vi "Running.vi"(8 "error in (no error)":errorcluster, 11 "CIFTemplatePlugin in":refnum<class "TemplatePlugin.lvclass">) -> (0 "error out":errorcluster, 2 "Destroy":bool, 3 "CIFTemplatePlugin out":refnum<class "TemplatePlugin.lvclass">)   [LabVIEW 2021, in "TemplatePlugin.lvclass"]
uses:
  TemplatePlugin.lvclass
  D:/dev/CIF-LVCore/src/CIFCore/Class/CIFCorePlugin.lvclass
  CIF-LVCore/src/CIFCore/Class/CIFCorePlugin.lvclass/CIFCorePlugin.ctl
  TemplatePlugin.lvclass/TemplatePlugin.ctl
  <vilib>/CIF Foundation/CIF Utilities/Statistics/I64/Stats_I64_CIF_U.lvclass/Stats_I64_CIF_U.ctl
  <vilib>/CIF Foundation/CIF Out of Band Commands/CIFOutOfBand.lvclass/CIFOutOfBand.ctl
  CIF-LVCore/src/Channels/CIFChannelMng/CIFChannelMng.lvclass/CIFChannelMng.ctl
  CIF-LVCore/src/CIFCore/OOB/OOB_Rx/CIFCoreOOB_Rx.lvclass/CIFCoreOOB_Rx.ctl
  <vilib>/CIF Foundation/CIF Channels Core/CIFChannels/CIFChannels.lvclass/CIFChannels.ctl
  CIF-LVCore/src/CIFCore/Class/Typedef/Energized States.ctl
  Logic.vi
  CIF-LVCore/src/CIFCore/Class/Accessors/Write Energized State.vi
  CIF-LVCore/src/CIFCore/Class/SubVIs/Sleep.vi
  CIF-LVCore/src/CIFCore/Class/SubVIs/Read Core OOB RX.vi
  gRPC/Read gRCP to Main.vi
  gRPC/Send Main to gRPC.vi
  CIF-LVCore/src/CIFCore/Class/SubVIs/OOB/Update Status from Benchmarks.vi
  CIF-LVCore/src/Channels/CIFChannelMng/Core/Send Channel List Update.vi
  <vilib>/CIF Foundation/CIF Utilities/Time/System Time/Sleep Until Future Time.vi
  <vilib>/CIF Foundation/CIF Utilities/Time/System Time/Get System Time.vi
  CIF-LVCore/src/CIFCore/Class/Channel RW/Read U64.vi
  CIF-LVCore/src/CIFCore/Class/Channel RW/Write U64.vi
  CIF-LVCore/src/CIFCore/Class/Channel RW/Read U8 Array FIFO.vi
  CIF-LVCore/src/CIFCore/Class/Channel RW/Write U8 Array FIFO.vi
  CIF-LVCore/src/CIFCore/Class/Channel RW/Write Double.vi
  CIF-LVCore/src/CIFCore/Class/Channel RW/Read Double.vi
  CIF-LVCore/src/CIFCore/Class/Accessors/Monitor/Write Double 1.vi
  CIF-LVCore/src/CIFCore/Class/Accessors/Monitor/Write U64 1.vi
  CIF-LVCore/src/CIFCore/Class/Accessors/Monitor/Write U64 2.vi
  CIF-LVCore/src/CIFCore/Class/Accessors/Monitor/Write I64 1.vi
  CIF-LVCore/src/CIFCore/Class/Accessors/Monitor/Write I64 2.vi
  CIF-LVCore/src/CIFCore/Class/Accessors/Timestamps/Write Execute TS.vi
  CIF-LVCore/src/CIFCore/Class/Accessors/Timestamps/Write Sleep TS.vi
  <vilib>/Utility/error.llb/Clear Errors.vi
  CIF-LVCore/src/CIFCore/Class/Accessors/Read Sleep Limits (ns).vi
  CIF-LVCore/src/CIFCore/Class/Accessors/Timestamps/Write Target Wake TS.vi
  CIF-LVCore/src/CIFCore/Common/Utilities/Add Error.vi
  CIF-LVCore/src/CIFCore/Class/Accessors/Read Plugin Name.vi
  CIF-LVCore/src/CIFCore/Class/Accessors/Timestamps/Read Running TS.vi
  CIF-LVCore/src/CIFCore/Class/Accessors/Read Running Internal Data.vi
  CIF-LVCore/src/CIFCore/Class/Accessors/Read Timing Override.vi
  CIF-LVCore/src/CIFCore/Class/Accessors/Read Common Config.vi
  CIF-LVCore/src/CIFCore/Class/Accessors/Timestamps/Write Housekeeping TS.vi
  <vilib>/CIF Foundation/CIF Utilities/Statistics/I64/X1 minus X0.vi
  <vilib>/CIF Foundation/CIF Utilities/Statistics/I64/Cyclic.vi
  CIF-LVCore/src/CIFCore/Class/Accessors/Timestamps/Read Execute TS.vi
  CIF-LVCore/src/CIFCore/Class/Accessors/Timestamps/Read Housekeeping TS.vi
  CIF-LVCore/src/CIFCore/Class/Accessors/Timestamps/Read Sleep TS.vi
  CIF-LVCore/src/CIFCore/Class/Accessors/Timestamps/Read Target Wake TS.vi
  CIF-LVCore/src/CIFCore/Class/SubVIs/Refresh Stats.vi
  CIF-LVCore/src/CIFCore/OOB/OOB_Rx/Receive/Read Clock Map.vi
  CIF-LVCore/src/Channels/CIFChannelMng/SubVIs/Connect Channel.vi
  CIF-LVCore/src/CIFCore/OOB/OOB_Rx/Receive/Read Connections.vi
  CIF-LVCore/src/CIFCore/OOB/OOB_Rx/Receive/Read Forces.vi
  CIF-LVCore/src/Channels/CIFChannelMng/SubVIs/Force Channel.vi
  CIF-LVCore/src/Channels/CIFChannelMng/SubVIs/Add FIFO Publisher.vi
  CIF-LVCore/src/CIFCore/OOB/OOB_Rx/Receive/Read Publisher Instance.vi
  CIF-LVCore/src/Channels/CIFChannelMng/Core/Send Publisher Instance Return.vi
  CIF-LVCore/src/Channels/CIFChannelMng/SubVIs/Remove FIFO Publisher.vi
  CIF-LVCore/src/CIFCore/OOB/OOB_Rx/Receive/Check for OOB Commands.vi
  OOB/OOB_Rx/Receive/Read Data.vi
  OOB/OOB_Rx/Receive/Check for OOB Commands.vi
  OOB/OOB_Tx/Send/Update Data.vi
  <vilib>/CIF Foundation/CIF Out of Band Commands/Commit Commands.vi
  CIF-LVCore/src/CIFCore/Class/Accessors/Read Refresh.vi
  <vilib>/CIF Foundation/CIF Utilities/Statistics/I64/Get Stats.vi
  CIF-LVCore/src/Channels/CIFChannelMng/OOB/OOB_Tx/Send/Update Channel List Command.vi
  <vilib>/CIF Foundation/CIF Utilities/Time/SubVIs/Add Error.vi
  <vilib>/CIF Foundation/CIF Utilities/Time/System Time/LabVIEW Time to TAI Time.vi
  <vilib>/CIF Foundation/CIF Utilities/Errors/Append Error Location.vi
  <vilib>/CIF Foundation/CIF Utilities/Statistics/I64/X1 minus X0.vi/dfabcf33-0dbc-4041-80a5-3dc0c86d2989.vi
  <vilib>/CIF Foundation/CIF Utilities/Statistics/I64/Cyclic.vi/dfabcf33-0dbc-4041-80a5-3dc0c86d2989.vi
  CIF-LVCore/src/CIFCore/OOB/OOB_Rx/Private/Read Payload.vi
  CIF-LVCore/src/Channels/CIFChannelMng/Utilities/Get Channel Index by Name.vi
  <vilib>/CIF Foundation/CIF Channels Core/CIFChannels/Accessors/Read Channel State.vi
  <vilib>/CIF Foundation/CIF Channels Core/CIFChannels/Accessors/Read Tag Forced.vi
  CIF-LVCore/src/Channels/CIFChannelMng/SubVIs/Add Error Channel Manager.vi
  CIF-LVCore/src/Channels/CIFChannelMng/OOB/OOB_Tx/Send/FIFO Publisher Return Command.vi
  CIF-LVCore/src/Channels/CIFChannelMng/SubVIs/Get Original FIFO Channel Name.vi
  <vilib>/CIF Foundation/CIF Out of Band Commands/Read Commands.vi
  CIF-LVCore/src/CIFCore/OOB/OOB_Rx/Private/Command Settings.vi
  OOB/OOB_Rx/Private/Read Payload.vi
  OOB/OOB_Rx/Private/Command Settings.vi
  <vilib>/CIF Foundation/CIF Out of Band Commands/Queue Command.vi
  <vilib>/CIF Foundation/CIF Out of Band Commands/Utilities/Command to Bitwise Command.vi
  <vilib>/CIF Foundation/CIF Out of Band Commands/Accessors/Read Local OOB Data.vi
  <vilib>/CIF Foundation/CIF Utilities/Statistics/I64/X1 minus X0.vi/dfabcf33-0dbc-4041-80a5-3dc0c86d2989.vi/9eb60a9a-770f-4d2d-8b3f-8465c267ecc9.vi
  <vilib>/CIF Foundation/CIF Utilities/Statistics/I64/Cyclic.vi/dfabcf33-0dbc-4041-80a5-3dc0c86d2989.vi/9eb60a9a-770f-4d2d-8b3f-8465c267ecc9.vi
  <vilib>/CIF Foundation/CIF Channels Core/ChannelCommon/Utilities/Add Error.vi
  OOB/OOB_Rx/TemplateOOB_Rx.lvclass
  C:/Program Files/National Instruments/LabVIEW 2021/vi.lib/CIF Foundation/CIF Out of Band Commands/CIFOutOfBand.lvclass
  OOB/OOB_Tx/TemplateOOB_Tx.lvclass
  CIF-LVCore/src/Channels/CIFChannelMng/OOB/OOB_Tx/ChnMngOOB_Tx.lvclass
  CIF-LVCore/src/CIFCore/OOB/OOB_Rx/CIFCoreOOB_Rx.lvclass
  <vilib>/CIF Foundation/CIF Channels Core/CIFChannels/Core/Set Force.vi
  <vilib>/CIF Foundation/CIF Channels Core/CIFChannels/CIFChannels.lvclass
  CIF-LVCore/src/CIFCore/Class/CIFCorePlugin.lvclass
  D:/dev/Plugins/Template/Class/TemplatePlugin.lvclass
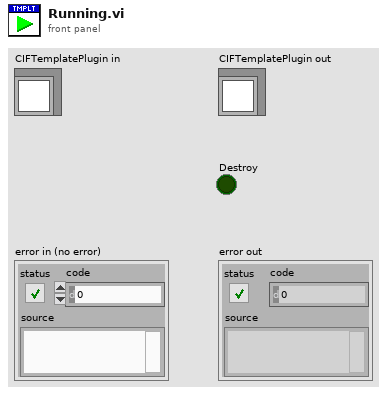
[diagram p1: front panel]
types:
  T1 = typedef "CIFCorePlugin.lvclass/Energized States.ctl" = enum16{"Listen", "Prepare", "Execute", "Housekeep", "Cleanup", "Destroy"}
  T2 = typedef "CIFCorePlugin.lvclass/Running State Logic.ctl" = enum16{"Execute", "Housekeep", "Cleanup", "Error", "Destroy"}
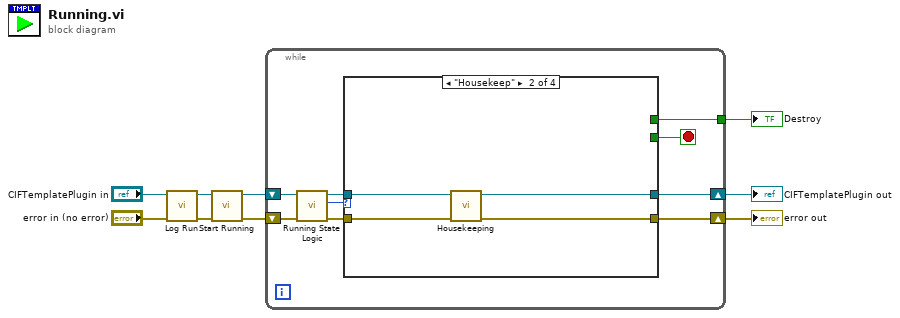
[diagram p0: block diagram]
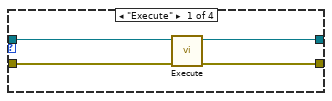
[diagram p2: hidden frame]
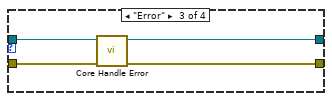
[diagram p3: hidden frame]
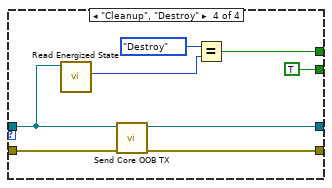
[diagram p4: hidden frame]
diagram:
  n1 = call "Log Run.vi"("error in (no error)"="error in (no error)", "CIFCorePlugin in"="CIFTemplatePlugin in") -> ("error out"=w8:errorcluster, "CIFCorePlugin out"=w9:refnum<class "TemplatePlugin.lvclass">)  [unwired: 8 in]
  n2 = call "Start Running.vi"("error in (no error)"=w8, "CIFCorePlugin in"=w9) -> ("error out"=w7:errorcluster, "CIFCorePlugin in"=w6:refnum<class "TemplatePlugin.lvclass">)  [unwired: 8 in]
  n3 = while {
    shift-right: [w13] -> w4
    shift-left: w6 -> [w18]
    shift-right: [w12] -> w5
    shift-left: w7 -> [w17]
    tunnel: [w10] -> w3
    stop <- w11 stop-if-true
    n4 = call "Running State Logic.vi"("error in (no error)"=w17, "CIFCorePlugin in"=w18) -> ("error out"=w14:errorcluster, "Running State Logic"=w16:T2, "CIFCorePlugin in"=w15:refnum<class "TemplatePlugin.lvclass">)  [unwired: 7 in]
    n5 = case shown="\"Housekeep\"" w16 {
      tunnel: w15 -> [w22 w26 w30 w32]
      tunnel: w14 -> [w21 w25 w29 w37]
      tunnel: [w20 w24 w28 w36] -> w13
      tunnel: [w19 w23 w27 w35] -> w12
      tunnel: [_ _ _ TRUE] -> w11
      tunnel: [_ _ _ w33] -> w10
      frame "Execute" {
        n6 = call "Execute.vi"("error in (no error)"=w21, "CIFTemplatePlugin in"=w22) -> ("error out"=w19:errorcluster, "CIFTemplatePlugin out"=w20:refnum<class "TemplatePlugin.lvclass">)  [unwired: 8 in]
      }
      frame "Housekeep" {
        n7 = call "Housekeeping.vi"("error in (no error)"=w25, "CIFTemplatePlugin in"=w26) -> ("error out"=w23:errorcluster, "CIFTemplatePlugin out"=w24:refnum<class "TemplatePlugin.lvclass">)  [unwired: 8 in]
      }
      frame "Error" {
        n8 = call "Core Handle Error.vi"("error in (no error)"=w29, "CIFTemplateNode in"=w30) -> ("error out"=w27:errorcluster, "CIFTemplateNode in"=w28:refnum<class "TemplatePlugin.lvclass">)  [unwired: 8 in]
      }
      frame "Cleanup", "Destroy" {
        n9 = call "Read Energized State.vi"("CIFCorePlugin in"=w32) -> ("Energized State"=w31:T1)  [unwired: 8 in, 2 out]
        n10 = call "Send Core OOB TX.vi"("error in (no error)"=w37, "CIFCorePlugin in"=w32) -> ("error out"=w35:errorcluster, "CIFCorePlugin in"=w36:refnum<class "TemplatePlugin.lvclass">)  [unwired: 8 in]
        n11 = Equal?(x=Energized_States."Destroy", y=w31) -> (x = y?=w33:bool)
      }
    }
  }
  "error out" <- w5
  "Destroy" <- w3
  "CIFTemplatePlugin out" <- w4
